vi "Inverse Kinematics.vi"(7 "Current Pod Steering (deg)":cluster{"LF":dbl, "LB":dbl, "RF":dbl, "RB":dbl}, 8 "Radii (ft)":T4 {"Right Back radius" format="%.2f"; "Right Front radius" format="%.2f"; "Left Back radius" format="%.2f"; "Left Front radius" format="%.2f"}, 9 "debug (F)":bool, 11 "Target Velocity (ft/s and deg/s)":cluster{"Vx":dbl, "Vy":dbl, "Omega":dbl}) -> (2 "Pod Setpoints (ft/s and deg)":T1, 4 "cross products":T2, 5 "A x B":T3, 6 "translation":dbl[](array[numeric]))   [LabVIEW 2020]
doc: "This VI calculates the velocity setpoints needed for the pods of a Swerve Drive. It takes in Robot centric velocities that describe the robot's motion, a cluster of the current orientations in degrees of each of the pods, and a cluster of the radius vectors from the center of mass to each of the swerve pods. It then outputs four clusters that represent the pod setpoints (velocity of the pod and orientation of the pod in ft/s and deg/s)\n\nOrder of all the clusters holding some kind of pod information will always be Left Front, Left Back, Right Front, Right Back"
uses:
  <vilib>/Analysis/Matrix/Datatypes/RealMatrix.ctl
  ctl/Pod Setpoints.ctl
  <vilib>/Analysis/coordinate.llb/Angle Range (Degree).ctl
  <vilib>/Analysis/coordinate.llb/Angle Units.ctl
  <vilib>/Analysis/coordinate.llb/Wrap Angle (scalar).vi
  <vilib>/Analysis/_algsub.llb/Real Vector Norm.vi
  <vilib>/Analysis/baseanly.llb/Real A x B.vi
  <vilib>/Analysis/Matrix/Numeric/Conversions/Array To Matrix - RA.vi
  <vilib>/Analysis/NI_AALPro.lvlib
  <vilib>/Analysis/Matrix/NI_Matrix.lvlib
  <vilib>/Analysis/NI_AALBase.lvlib
  <vilib>/Analysis/NI_AAL_Angle.lvlib
panel:
  # "Diganostics for the Visualizer"
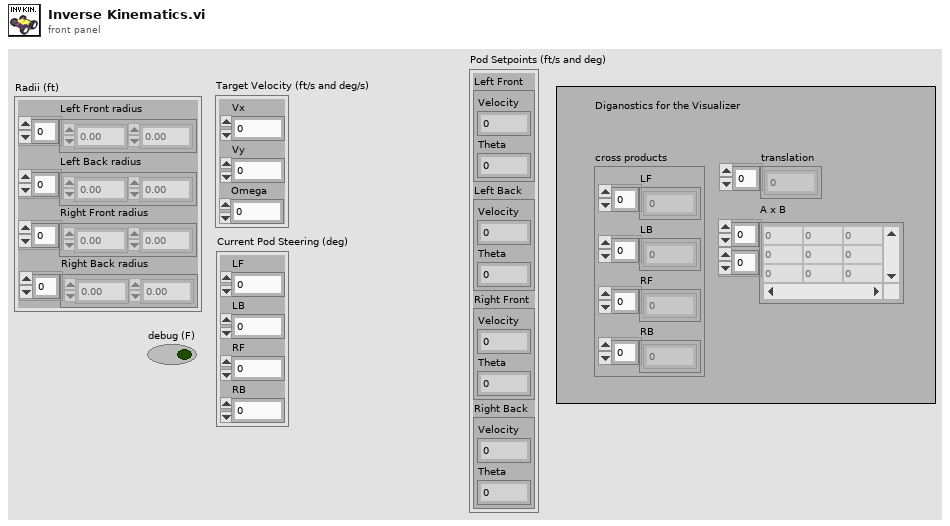
[diagram p1: front panel]
types:
  T1 = typedef "Pod Setpoints.ctl" = cluster{"Left Front":cluster{"Velocity":dbl, "Theta":dbl}, "Left Back":cluster{"Velocity":dbl, "Theta":dbl}, "Right Front":cluster{"Velocity":dbl, "Theta":dbl}, "Right Back":cluster{"Velocity":dbl, "Theta":dbl}}
  T2 = cluster{"LF":dbl[], "LB":dbl[], "RF":dbl[], "RB":dbl[]}
  T3 = typedef "NI_Matrix.lvlib/RealMatrix.ctl" = dbl[][]
  T4 = cluster{"Left Front radius":dbl[], "Left Back radius":dbl[], "Right Front radius":dbl[], "Right Back radius":dbl[]}
  T5 = typedef "NI_AAL_Angle.lvlib/Angle Units.ctl" = i32
  T6 = typedef "NI_AAL_Angle.lvlib/Angle Range (Degree).ctl" = u16
  T7 = cluster{"new v + travel":cluster{"velocity":dbl, "travel angle":dbl}, "new v + travel":cluster{"velocity":dbl, "travel angle":dbl}, "new v + travel":cluster{"velocity":dbl, "travel angle":dbl}, "new v + travel":cluster{"velocity":dbl, "travel angle":dbl}}
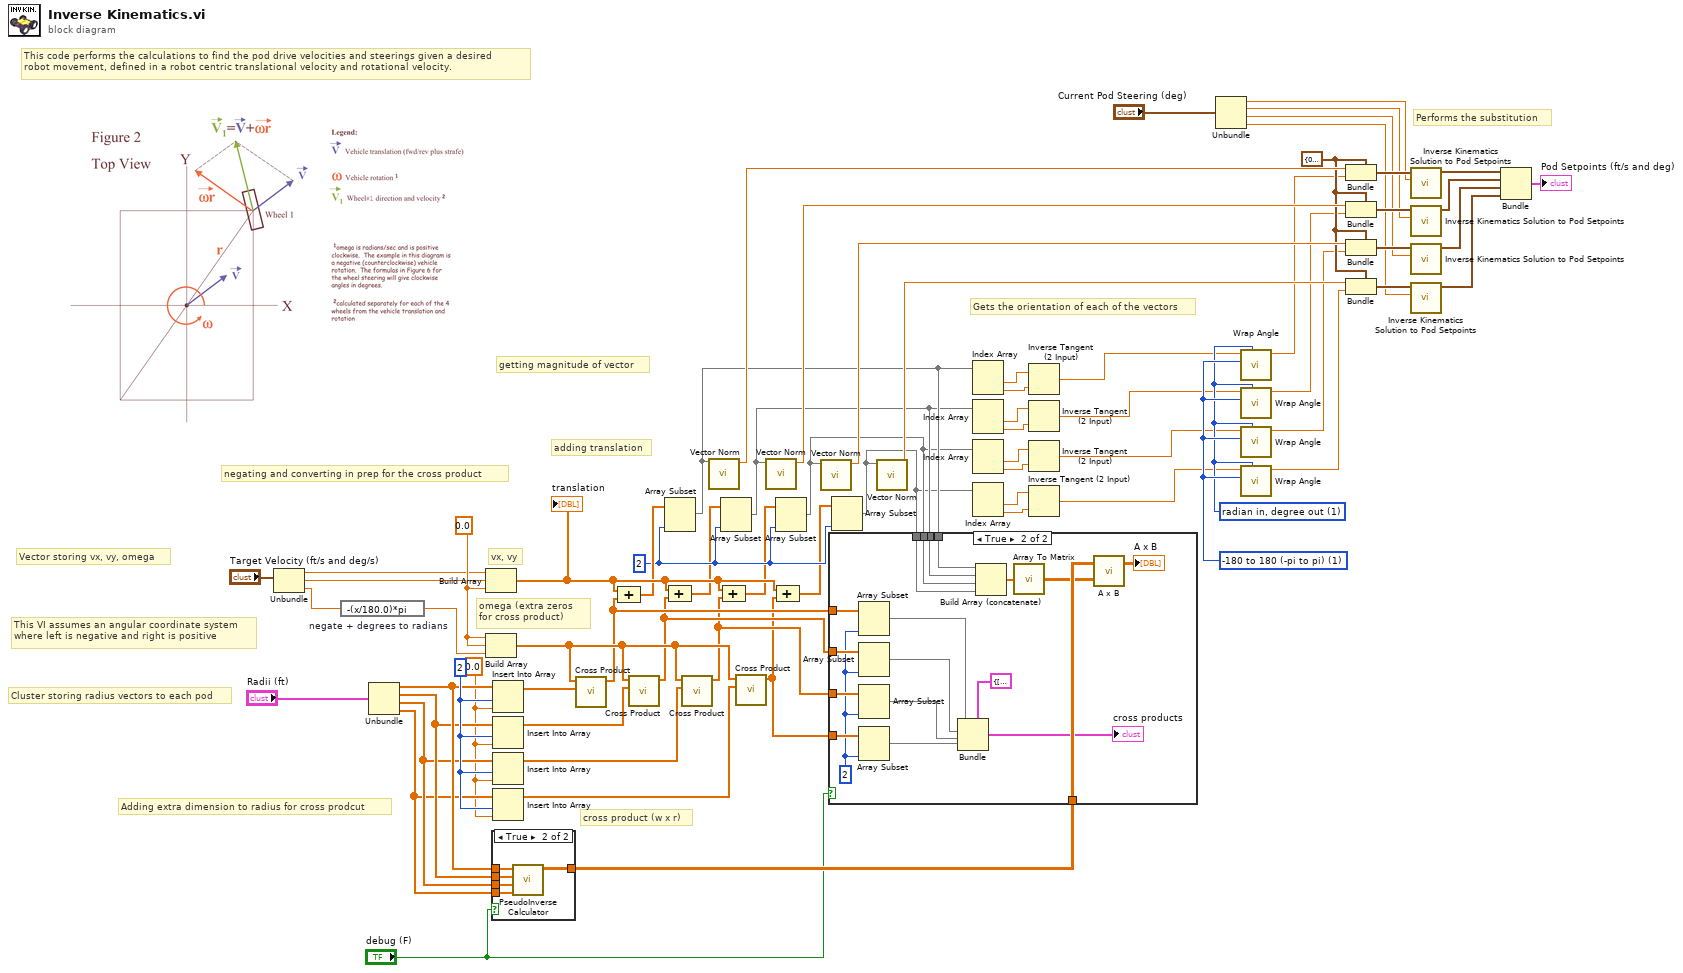
[diagram p0: block diagram]
diagram:
  w23 = 0.0 ("new element/subarray")
  w24 = T5 1 items=["radian in, radian out", "radian in, degree out", "degree in, degree out", "degree in, radian out"] ("angle units")
  w25 = T6 1 items=["none", "-180 to 180 (-pi to pi)", "0 to 360 (0 to 2pi)"] ("angle range")
  w57 = 2 ("index")
  w58 = cluster{"Velocity":dbl, "Theta":dbl} {"Velocity"=0.0, "Theta"=0.0} ("Pod Setpoints")
  w66 = 2 ("length")
  w71 = 0.0 ("element")
  # "This code performs the calculations to find the pod drive velocities and steerings given a desired\nrobot movement, defined in a robot centric translational velocity and rotational velocity."
  # "Performs the substitution"
  # "Gets the orientation of each of the vectors"
  # "getting magnitude of vector"
  # "adding translation"
  # "cross product (w x r)"
  # "Adding extra dimension to radius for cross prodcut"
  # "negating and converting in prep for the cross product"
  # "This VI assumes an angular coordinate system\nwhere left is negative and right is positive"
  # "omega (extra zeros for cross product)"
  # "vx, vy"
  # "Cluster storing radius vectors to each pod"
  # "Vector storing vx, vy, omega"
  n1 = Unbundle("Target Velocity (ft/s and deg/s)") -> ("Vx"=w33:dbl, "Vy"=w32:dbl, "Omega"=w26:dbl)
  n2 = expression code="-(x/180.0)*pi" "negate + degrees to radians"(w26) -> (w52:dbl)
  n3 = Unbundle("Radii (ft)") -> ("Left Front radius"=w51:dbl[], "Left Back radius"=w50:dbl[], "Right Front radius"=w49:dbl[], "Right Back radius"=w48:dbl[])
  n4 = Build Array(w33, w32, w71) -> (w68:dbl[])
  "translation" <- w68
  n5 = Build Array(w71, w71, w52) -> (w69:dbl[])
  n6 = case shown="True" "debug (F)" {
    tunnel: w51 -> [_ w76]
    tunnel: w50 -> [_ w75]
    tunnel: w49 -> [_ w74]
    tunnel: w48 -> [_ w73]
    tunnel: [_ w72] -> w47
    frame False {
    }
    frame True {
      n7 = call "PseudoInverse Calculator.vi"("R4"=w73, "R3"=w74, "R2"=w75, "R1"=w76) -> ("Pseudoinverse"=w72:T3)  [unwired: 7 in]
    }
  }
  n8 = Insert Into Array(array=w51, index=w57, new element=w23) -> (w56:dbl[])
  n9 = Insert Into Array(array=w50, index=w57, new element=w23) -> (w55:dbl[])
  n10 = Insert Into Array(array=w49, index=w57, new element=w23) -> (w54:dbl[])
  n11 = Insert Into Array(array=w48, index=w57, new element=w23) -> (w53:dbl[])
  n12 = call <vilib>:"Cross Product.vi"("B Vector"=w56, "A Vector"=w69) -> ("Cross Product"=w46:dbl[])  [unwired: 8 in, 1 out]
  n13 = Compound Arithmetic op=ADD(w68, w46) -> (w67:dbl[])
  n14 = call <vilib>:"Cross Product.vi"("B Vector"=w55, "A Vector"=w69) -> ("Cross Product"=w45:dbl[])  [unwired: 8 in, 1 out]
  n15 = Array Subset(array=w67, length=w66) -> (w21:dbl[])  [unwired: 1 in]
  n16 = Compound Arithmetic op=ADD(w68, w45) -> (w65:dbl[])
  n17 = call <vilib>:"Cross Product.vi"("B Vector"=w54, "A Vector"=w69) -> ("Cross Product"=w44:dbl[])  [unwired: 8 in, 1 out]
  n18 = call-poly <vilib>:"Vector Norm.vi"("Input Vector"=w21) -> ("norm"=w62:dbl)  [unwired: 9 in, 1 out]
  n19 = Array Subset(array=w65, length=w66) -> (w18:dbl[])  [unwired: 1 in]
  n20 = Compound Arithmetic op=ADD(w68, w44) -> (w64:dbl[])
  n21 = call <vilib>:"Cross Product.vi"("B Vector"=w53, "A Vector"=w69) -> ("Cross Product"=w43:dbl[])  [unwired: 8 in, 1 out]
  n22 = call-poly <vilib>:"Vector Norm.vi"("Input Vector"=w18) -> ("norm"=w61:dbl)  [unwired: 9 in, 1 out]
  n23 = Array Subset(array=w64, length=w66) -> (w13:dbl[])  [unwired: 1 in]
  n24 = Compound Arithmetic op=ADD(w68, w43) -> (w63:dbl[])
  n25 = call-poly <vilib>:"Vector Norm.vi"("Input Vector"=w13) -> ("norm"=w60:dbl)  [unwired: 9 in, 1 out]
  n26 = Array Subset(array=w63, length=w66) -> (w12:dbl[])  [unwired: 1 in]
  n27 = case shown="True" "debug (F)" {
    tunnel: w21 -> [_ w95]
    tunnel: w18 -> [_ w94]
    tunnel: w13 -> [_ w93]
    tunnel: w12 -> [_ w92]
    tunnel: w47 -> [_ w91]
    tunnel: w46 -> [_ w90]
    tunnel: w45 -> [_ w89]
    tunnel: w44 -> [_ w88]
    tunnel: w43 -> [_ w87]
    frame False {
    }
    frame True {
      w77 = 2 ("length")
      n28 = Array Subset(array=w90, length=w77) -> (w86:dbl[])  [unwired: 1 in]
      n29 = Array Subset(array=w89, length=w77) -> (w85:dbl[])  [unwired: 1 in]
      n30 = Array Subset(array=w88, length=w77) -> (w84:dbl[])  [unwired: 1 in]
      n31 = Array Subset(array=w87, length=w77) -> (w83:dbl[])  [unwired: 1 in]
      n32 = Bundle(cluster=T2 {"LF"=[], "LB"=[], "RF"=[], "RB"=[]}, "LF"=w86, "LB"=w85, "RF"=w84, "RB"=w83) -> (→"cross products":T2)
      n33 = Build Array (concatenate)(w95, w94, w93, w92) -> (w80:dbl[])
      n34 = call-poly <vilib>:"Array To Matrix.vi"("Real 1D Array"=w80) -> ("Real Matrix (Column Vector)"=w78:T3)
      n35 = call-poly <vilib>:"A x B.vi"("B"=w78, "A"=w91) -> ("A x B"=→"A x B":T3)  [unwired: 1 out]
    }
  }
  n36 = call-poly <vilib>:"Vector Norm.vi"("Input Vector"=w12) -> ("norm"=w59:dbl)  [unwired: 9 in, 1 out]
  n37 = Index Array(array=w21) -> (element #1=w20:dbl, element #2=w19:dbl)  [unwired: 2 in]
  n38 = Index Array(array=w18) -> (element #1=w17:dbl, element #2=w16:dbl)  [unwired: 2 in]
  n39 = Index Array(array=w13) -> (element #1=w10:dbl, element #2=w11:dbl)  [unwired: 2 in]
  n40 = Index Array(array=w12) -> (element #1=w9:dbl, element #2=w8:dbl)  [unwired: 2 in]
  n41 = Inverse Tangent (2 Input)(1:w19, 2:w20) -> (0:w15:dbl)
  n42 = Inverse Tangent (2 Input)(1:w16, 2:w17) -> (0:w14:dbl)
  n43 = Inverse Tangent (2 Input)(1:w11, 2:w10) -> (0:w7:dbl)
  n44 = Inverse Tangent (2 Input)(1:w8, 2:w9) -> (0:w6:dbl)
  n45 = Unbundle("Current Pod Steering (deg)") -> ("LF"=w30:dbl, "LB"=w29:dbl, "RF"=w28:dbl, "RB"=w27:dbl)
  n46 = call-poly <vilib>:"Wrap Angle.vi"("angle units"=w24, "angle range"=w25, "angle in"=w15) -> ("angle out"=w42:dbl)  [unwired: 7 in, 1 out]
  n47 = call-poly <vilib>:"Wrap Angle.vi"("angle units"=w24, "angle range"=w25, "angle in"=w14) -> ("angle out"=w41:dbl)  [unwired: 7 in, 1 out]
  n48 = call-poly <vilib>:"Wrap Angle.vi"("angle units"=w24, "angle range"=w25, "angle in"=w7) -> ("angle out"=w40:dbl)  [unwired: 7 in, 1 out]
  n49 = call-poly <vilib>:"Wrap Angle.vi"("angle units"=w24, "angle range"=w25, "angle in"=w6) -> ("angle out"=w39:dbl)  [unwired: 7 in, 1 out]
  n50 = Bundle(cluster=w58, "Velocity"=w62, "Theta"=w42) -> (w38:cluster{"Velocity":dbl, "Theta":dbl})
  n51 = Bundle(cluster=w58, "Velocity"=w61, "Theta"=w41) -> (w37:cluster{"Velocity":dbl, "Theta":dbl})
  n52 = Bundle(cluster=w58, "Velocity"=w60, "Theta"=w40) -> (w36:cluster{"Velocity":dbl, "Theta":dbl})
  n53 = Bundle(cluster=w58, "Velocity"=w59, "Theta"=w39) -> (w35:cluster{"Velocity":dbl, "Theta":dbl})
  n54 = call "Inverse Kinematics Solution to Pod Setpoints.vi"("actual theta"=w30, "v + target"=w38) -> ("new v + travel"=w5:cluster{"velocity":dbl, "travel angle":dbl})  [unwired: 9 in]
  n55 = call "Inverse Kinematics Solution to Pod Setpoints.vi"("actual theta"=w29, "v + target"=w37) -> ("new v + travel"=w4:cluster{"velocity":dbl, "travel angle":dbl})  [unwired: 9 in]
  n56 = call "Inverse Kinematics Solution to Pod Setpoints.vi"("actual theta"=w28, "v + target"=w36) -> ("new v + travel"=w3:cluster{"velocity":dbl, "travel angle":dbl})  [unwired: 9 in]
  n57 = call "Inverse Kinematics Solution to Pod Setpoints.vi"("actual theta"=w27, "v + target"=w35) -> ("new v + travel"=w2:cluster{"velocity":dbl, "travel angle":dbl})  [unwired: 9 in]
  n58 = Bundle("new v + travel"=w5, "new v + travel"=w4, "new v + travel"=w3, "new v + travel"=w2) -> (→"Pod Setpoints (ft/s and deg)":T7)  [unwired: 1 in]
